vi "Initialize.vi"(8 "error in (no error)":errorcluster, 10 "Device":string) -> (0 "error out":errorcluster, 3 "Robot out":refnum<class "Robot.lvclass">)   [LabVIEW 2018, in "Robot.lvlib" / "Robot.lvclass"]
uses:
  Robot.lvclass
  Robot.lvclass/Robot.ctl
  PPLs/Configuration/Configuration.lvlibp/Configuration.lvclass
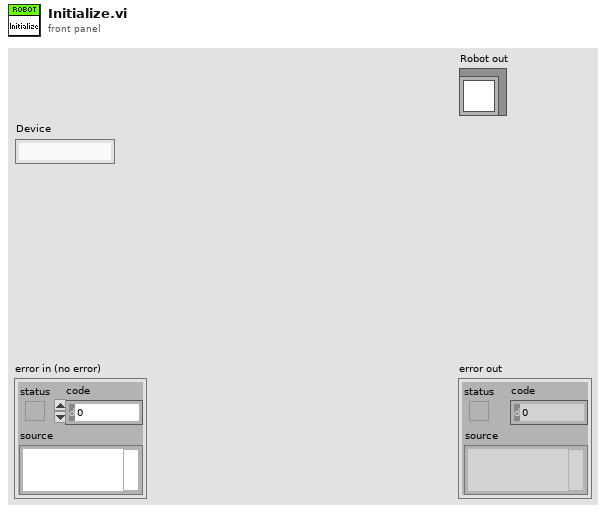
[diagram p1: front panel]
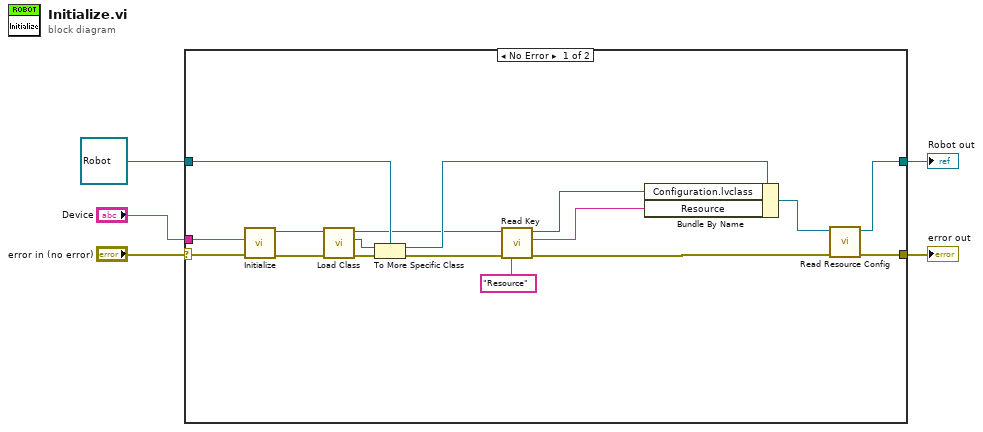
[diagram p0: block diagram]
diagram:
  n1 = case shown="No Error" "error in (no error)" {
    selector: "error in (no error)" -> [w21 w24]
    tunnel: [w8 w24] -> w4
    tunnel: [w6 w23] -> w1
    tunnel: "Device" -> [w22 _]
    tunnel: refnum<class "Robot.lvclass"> refnum ("Robot.lvlib:Robot.lvclass") -> [w16 w23]
    frame No Error {
      n2 = call "Initialize.vi"("error in"=w21, "Device"=w22) -> ("error out"=w19:errorcluster, "Configuration out"=w20:refnum<class "Configuration.lvclass">)  [unwired: 8 in]
      n3 = call "Load Class.vi"("error in"=w19, "Configuration in"=w20) -> ("error out"=w18:errorcluster, "Class out"=w17:refnum<class>, "Configuration out"=w13:refnum<class "Configuration.lvclass">)  [unwired: 7 in]
      n4 = To More Specific Class(target class=w16, reference=w17, error in=w18) -> (specific class reference=w14:refnum<class "Robot.lvclass">, error out=w15:errorcluster)
      n5 = call "Read Key.vi"("Key:"="Resource", "error in"=w15, "Configuration in"=w13) -> ("error out"=w9:errorcluster, "Value"=w11:string, "Configuration out"=w10:refnum<class "Configuration.lvclass">)  [unwired: 6 in]
      n6 = Bundle By Name(cluster=w14, "Configuration.lvclass"=w10, "Resource"=w11) -> (w7:refnum<class "Robot.lvclass">)
      n7 = call "Read Resource Config.vi"("error in (no error)"=w9, "Robot.lvclass"=w7) -> ("error out"=w8:errorcluster, "Robot.lvclass"=w6:refnum<class "Robot.lvclass">)  [unwired: 8 in]
    }
    frame Error {
    }
  }
  "error out" <- w4
  "Robot out" <- w1
